vi "Read Message Priority.vi"(8 "error in (no error)":errorcluster, 11 "Publisher Msg in":refnum<class "Publisher Msg.lvclass">) -> (0 "error out":errorcluster, 2 "Message Priority":T1=enum."Normal", 3 "Publisher Msg out":refnum<class "Publisher Msg.lvclass">)   [LabVIEW 2020, in "Publisher.lvlib" / "Publisher Msg.lvclass"]
uses:
  Publisher Msg.lvclass
  PPL/HDH.Actor Framework.Core.Actor.lvlibp/1abvi3w/vi.lib/ActorFramework/Message Enqueuer/Message Priority.ctl
  Publisher Msg.lvclass/Publisher Msg.ctl
  PPL/HDH.Actor Framework.Core.Actor.lvlibp/1abvi3w/vi.lib/ActorFramework/Message Enqueuer/Message Enqueuer.lvclass
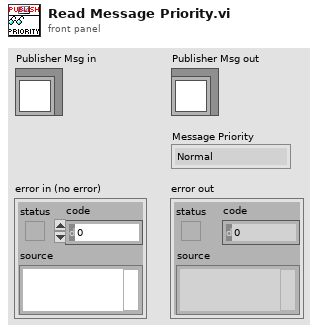
[diagram p1: front panel]
types:
  T1 = typedef "HDH.Actor Framework.Core.Actor.lvlibp/Message Enqueuer.lvclass/Message Priority.ctl" = enum16{"Low", "Normal", "High"}
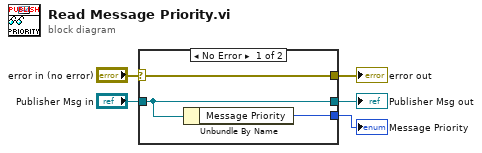
[diagram p0: block diagram]
diagram:
  n1 = case shown="No Error" "error in (no error)" {
    selector: "error in (no error)" -> [w8 w9]
    tunnel: [w8 w9] -> w4
    tunnel: [w7 w10] -> w2
    tunnel: "Publisher Msg in" -> [w7 w10]
    tunnel: [w6 _] -> w1
    frame No Error {
      n2 = Unbundle By Name(w7) -> ("Message Priority"=w6:T1)
    }
    frame Error {
    }
  }
  "error out" <- w4
  "Publisher Msg out" <- w2
  "Message Priority" <- w1
